vi "angle_corrector2.vi"(10 "angle":dbl) -> (2 "angle corrected":dbl)   [LabVIEW 2020]
panel:
  out "# ciclos":i32
  # "Angle corrector"
  # "com detector de ciclos"
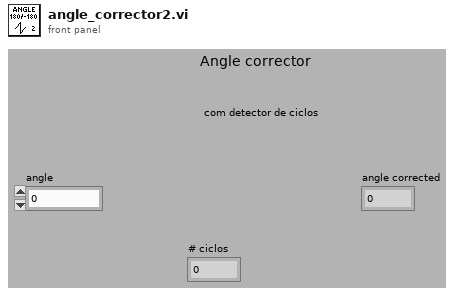
[diagram p1: front panel]
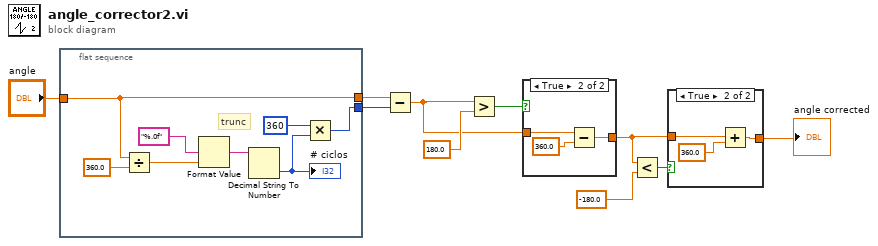
[diagram p0: block diagram]
diagram:
  n1 = flat-sequence {
    tunnel: [w14] -> w1
    tunnel: "angle" -> [w13]
    tunnel: [w13] -> w2
    frame #0 {
      # "trunc"
      n2 = Divide(x=w13, y=360.0) -> (x/y=w17:dbl)
      n3 = Format Value(format string="%.0f", value (0)=w17) -> (output string=w12:string)  [unwired: 1 in]
      n4 = Decimal String To Number(string=w12) -> (number=w16:i32)  [unwired: 2 in, 1 out]
      "# ciclos" <- w16
      n5 = Multiply(x=360, y=w16) -> (x*y=w14:i32)
    }
  }
  n6 = Subtract(x=w2, y=w1) -> (x-y=w4:dbl)
  n7 = Greater?(x=w4, y=180.0) -> (0:w8:bool)
  n8 = case shown="True" w8 {
    tunnel: w4 -> [w19 w21]
    tunnel: [w19 w20] -> w6
    frame False {
    }
    frame True {
      n9 = Subtract(x=w21, y=360.0) -> (x-y=w20:dbl)
    }
  }
  n10 = Less?(x=w6, y=-180.0) -> (x < y?=w7:bool)
  n11 = case shown="True" w7 {
    tunnel: w6 -> [w23 w25]
    tunnel: [w23 w24] -> w5
    frame False {
    }
    frame True {
      n12 = Add(x=w25, y=360.0) -> (x+y=w24:dbl)
    }
  }
  "angle corrected" <- w5
